vi "Add Connection to State.vi"(8 "error in (no error)":errorcluster, 10 "Connection":T1, 11 "Routing State in":T2) -> (0 "error out":errorcluster, 1 "already exists":bool, 3 "Routing State out":T2)   [LabVIEW 2017, in "Switch Scripting.lvlib"]
uses:
  Switch Scripting.lvlib
  Routing State.ctl
  Connection.ctl
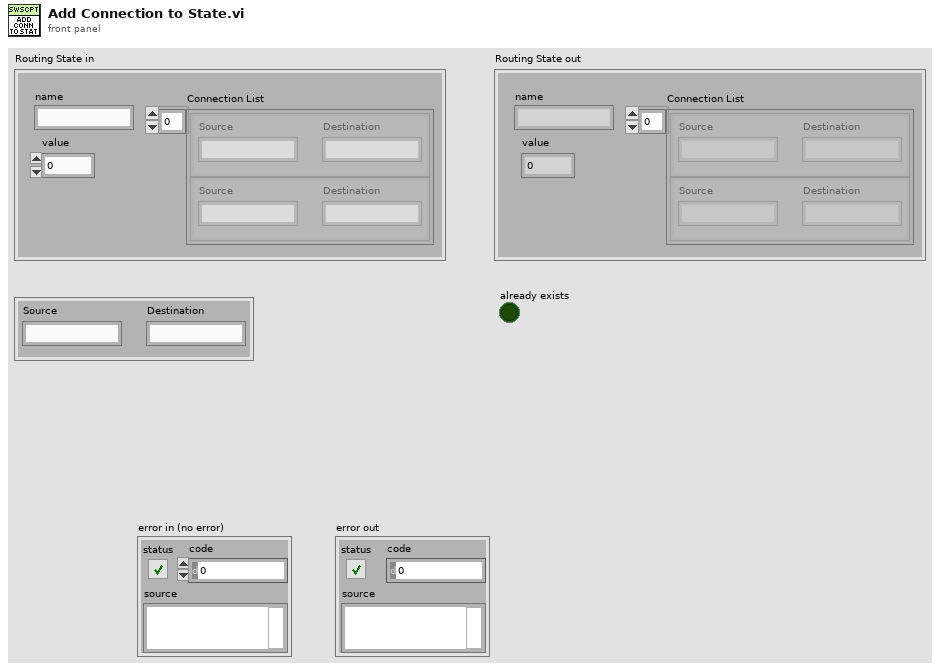
[diagram p1: front panel]
types:
  T1 = typedef "Switch Scripting.lvlib/Connection.ctl" = cluster{"Source":string, "Destination":string}
  T2 = typedef "Switch Scripting.lvlib/Routing State.ctl" = cluster{"name":string, "value":i32, "Connection List":T1[]}
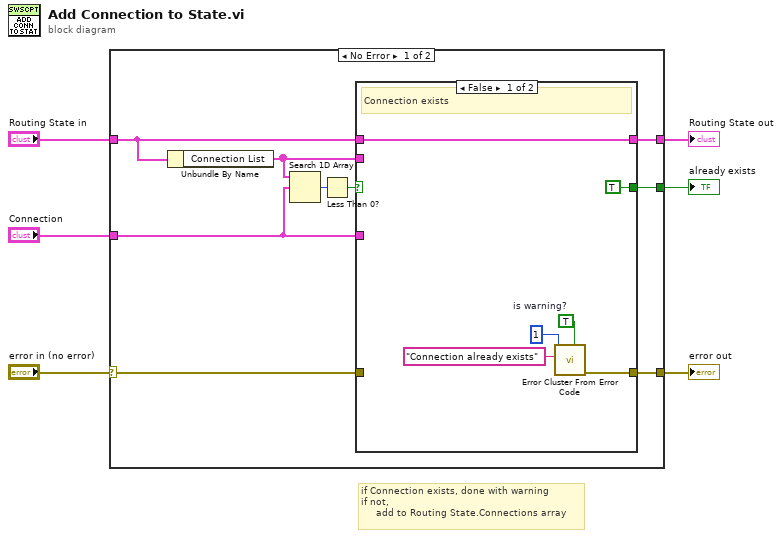
[diagram p0: block diagram]
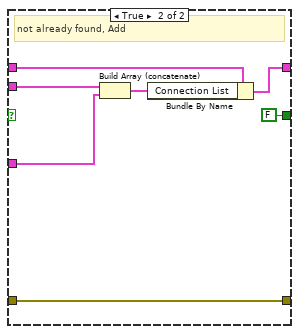
[diagram p2: hidden frame]
diagram:
  # "if Connection exists, done with warning\nif not, \n     add to Routing State.Connections array"
  n1 = case shown="No Error" "error in (no error)" {
    selector: "error in (no error)" -> [w15 w30]
    tunnel: [w14 w30] -> w6
    tunnel: [w7 w29] -> w5
    tunnel: "Routing State in" -> [w8 w29]
    tunnel: "Connection" -> [w9 _]
    tunnel: [w11 _] -> w1
    frame No Error {
      n2 = Unbundle By Name(w8) -> ("Connection List"=w10:T1[])
      n3 = Search 1D Array(1D array=w10, element=w9) -> (index of element=w13:i32)  [unwired: 1 in]
      n4 = Less Than 0?(x=w13) -> (x < 0?=w12:bool)
      n5 = case shown="False" w12 {
        tunnel: w15 -> [_ w28]
        tunnel: [w19 w28] -> w14
        tunnel: [TRUE FALSE] -> w11
        tunnel: w10 -> [_ w26]
        tunnel: w9 -> [_ w25]
        tunnel: w8 -> [w18 w24]
        tunnel: [w18 w22] -> w7
        frame False {
          w20 = TRUE  # is warning?
          # "Connection exists"
          n6 = call <vilib>:"Error Cluster From Error Code.vi"("is warning? (False)"=w20, "error message (\"\")"="Connection already exists" ("error message (\"\")"), "error code (0)"=1) -> ("error out"=w19:errorcluster)  [unwired: 6 in]
        }
        frame True {
          # "not already found, Add"
          n7 = Build Array (concatenate)(w26, w25) -> (w23:T1[])
          n8 = Bundle By Name(cluster=w24, "Connection List"=w23) -> (w22:T2)
        }
      }
    }
    frame Error {
    }
  }
  "error out" <- w6
  "Routing State out" <- w5
  "already exists" <- w1
